vi "DAQmx Create AI Channel TEDS(sub).vi"(0 "task in":refnum<k21>, 1 "virtual channel name":string, 5 "physical channel name":tag, 7 "measurement type":i32(ring)=10322 items=["Voltage"=10322, "Current"=10134, "More:Voltage:Custom with Excitation"=10323, "More:Current:Custom with Excitation"=10136, "Frequency"=10181, "Period"=10257, "Resistance"=10278, "Temperature:Thermocouple"=10303, "Temperature:Thermistor"=10302, "Temperature:RTD"=10301, "Temperature:Built-in Sensor"=10311, "Strain Gage"=10300, "LVDT"=10352, "RVDT"=10353, "Accelerometer:Voltage Input"=10355, "Accelerometer:Current Input"=10356, "Sound Pressure:Microphone"=10354, "TEDS"=12531], 11 "error in":errorcluster, 13 "custom scale":tag) -> (4 "task out":refnum<k21>, 6 "channel names":string, 15 "error out":errorcluster)   [LabVIEW 2011]
uses:
  nilvaiu.dll
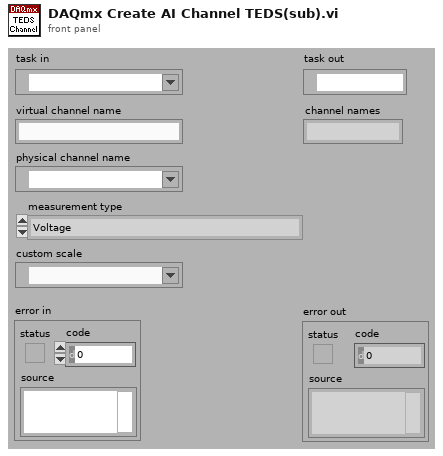
[diagram p1: front panel]
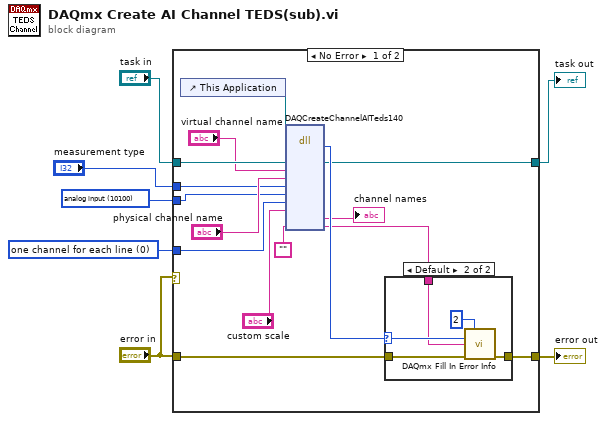
[diagram p0: block diagram]
diagram:
  w3 = 0 items=["one channel for each line", "one channel for all lines"] ("line grouping")
  w4 = 10100 items=["analog input"=10100, "analog output"=10102, "digital input"=10151, "digital output"=10153, "counter input"=10131, "counter output"=10132] ("channel type")
  n1 = case shown="No Error" "error in" {
    tunnel: [w20 w30] -> w7
    tunnel: "error in" -> [w22 w30]
    tunnel: "task in" -> [w18 w29]
    tunnel: "measurement type" -> [w15 _]
    tunnel: w4 -> [w14 _]
    tunnel: w3 -> [w13 _]
    tunnel: [w8 w29] -> w1
    frame No Error {
      n2 = control-ref of="This Application"() -> (w9:refnum<vi>)
      n3 = dll-call lib="nilvaiu.*" fn="DAQCreateChannelAITeds140"("This Application"=w9, "task in"=w18, "virtual channel name"="virtual channel name", "physical channel name"="physical channel name", "measurement type"=w15, "channel type"=w14, "line grouping"=w13, "customScale"="custom scale", "extendedErrorIndo"="") -> (w21:i32, "task in"=w8:refnum<k21>, "channel names"=→"channel names":string, "extendedErrorIndo"=w10:string)  [unwired: 10 in, 3 out]
      n4 = case shown="Default" w21 {
        selector: w21 -> [_ w26]
        tunnel: w22 -> [w23 w28]
        tunnel: [w23 w27] -> w20
        tunnel: w10 -> [_ w24]
        frame 0 {
        }
        frame Default {
          n5 = call "DAQmx Fill In Error Info.vi"("depth"=2, "status code"=w26, "extended error info"=w24, "error in"=w28) -> ("error out"=w27:errorcluster)  [unwired: 1 in, 10 out]
        }
      }
    }
    frame Error {
    }
  }
  "error out" <- w7
  "task out" <- w1
